vi "ACIR Instrument UI.vi"() -> ()   [LabVIEW 2025, in "ACIR.lvlib" / "ACIR Instrument.lvclass"]
doc: "Copyright 2017 National Instruments Corporation\n\nLicensed under the Apache License, Version 2.0 (the \"License\"); you may not use this file except in compliance with the License. You may obtain a copy of the License at http://www.apache.org/licenses/LICENSE-2.0\nUnless required by applicable law or agreed to in writing, software distributed under the License is distributed on an \"AS IS\" BASIS, WITHOUT WARRANTIES OR CONDITIONS OF ANY KIND, either express or implied. See the License for the specific language governing permissions and limitations under the License."
uses:
  ACIR Instrument.lvclass
  Users/Public/Documents/Sandia National Labs/TSS Plugin/CEF.lvlibp/Node/NodeRef.ctl
  Users/Public/Documents/Sandia National Labs/TSS Plugin/CEF.lvlibp/Node/CEF_Node.lvclass
  Users/Public/Documents/Sandia National Labs/TSS Plugin/CEF.lvlibp/Node/mainQref.ctl
  Users/Public/Documents/Sandia National Labs/TSS Plugin/CEF.lvlibp/Node/UserEventRef.ctl
  Users/Public/Documents/Sandia National Labs/TSS Plugin/Abstract Engine.lvlibp/Instrument configuration/Default Instrument.ctl
  ACIR configuration/ACIR Instrument Setting.ctl
  C:/Users/Public/Documents/Sandia National Labs/TSS Plugin/CEF.lvlibp/Node/CEF_Node.lvclass
  ACIR Instrument.lvclass/ACIR Instrument.ctl
  ACIR configuration/ACIR configuration.lvclass/ACIR configuration.ctl
  ACIR configuration/Read ACIR Setting.vi
  ACIR configuration/Write ACIR Setting.vi
  <vilib>/Utility/error.llb/Trim Whitespace One-Sided.vi
  ACIR configuration/ACIR configuration.lvclass
  C:/Users/Public/Documents/Sandia National Labs/TSS Plugin/Abstract Engine.lvlibp/Instrument configuration/Instrument configuration.lvclass
  Users/Public/Documents/Sandia National Labs/TSS Plugin/Abstract Engine.lvlibp/Instrument configuration/Read Instrument Setting.vi
  Users/Public/Documents/Sandia National Labs/TSS Plugin/Abstract Engine.lvlibp/Instrument configuration/Write Instrument Setting.vi
  Users/Public/Documents/Sandia National Labs/TSS Plugin/Abstract Engine.lvlibp/Instrument configuration/Instrument configuration.lvclass
panel:
  in  "ACIR":cluster{"Default":T1, "Setting":T2}={"Default"={"Type"="NI Digitizer", "Address"="None", "SW Alias"="None", "Description"="* Type = Class\n\n** Concrete = Specific  Device\nConcreate should be same with Type\n ", "Enabled"=TRUE}, "Setting"={"Frequency"=0.0, "Range"="100m Ohm", "Measurements"="Impedence"}} {"Setting"."Frequency" format="%#_6p"}
  in  "user event":T3
  in  "main queue":T4
  in  "node ref":T5
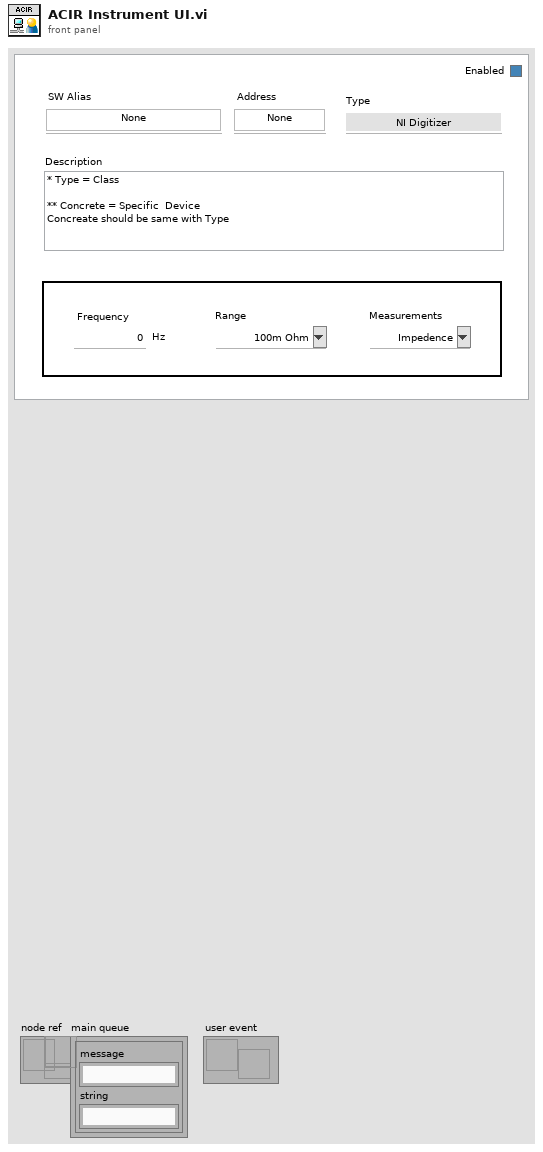
[diagram p1: front panel]
types:
  T1 = typedef "Abstract Engine.lvlibp/Instrument configuration.lvclass/Default Instrument.ctl" = cluster{"Type":string, "Address":string, "SW Alias":string, "Description":string, "Enabled":bool}
  T2 = typedef "ACIR.lvlib/ACIR configuration.lvclass/ACIR Instrument Setting.ctl" = cluster{"Frequency":dbl, "Range":string, "Measurements":string}
  T3 = typedef "CEF.lvlibp/CEF_Node.lvclass/UserEventRef.ctl" = refnum<user-event>
  T4 = typedef "CEF.lvlibp/CEF_Node.lvclass/mainQref.ctl" = refnum<queue>
  T5 = typedef "CEF.lvlibp/CEF_Node.lvclass/NodeRef.ctl" = refnum<data-value>
  T6 = cluster{"Instrument Setting":T1, "ACIR Setting":T2}
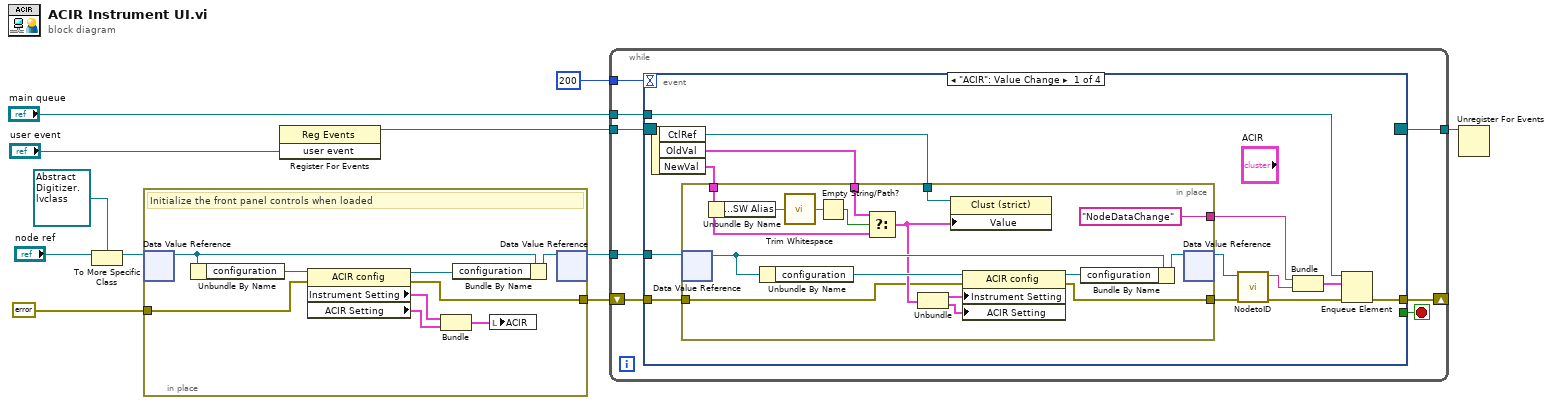
[diagram p0: block diagram]
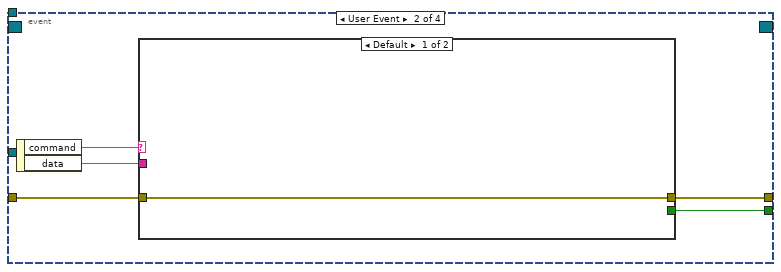
[diagram p2: hidden frame]
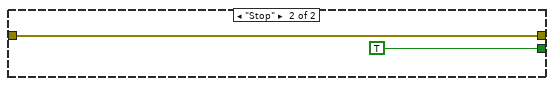
[diagram p3: hidden frame]
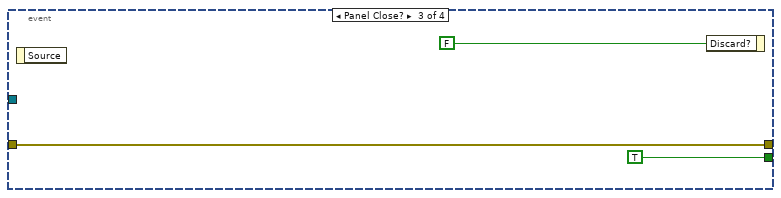
[diagram p4: hidden frame]
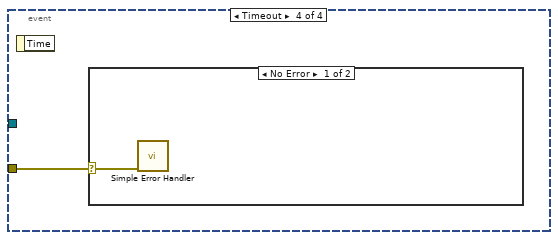
[diagram p5: hidden frame]
diagram:
  n1 = To More Specific Class(target class=refnum<data-value> refnum ("data value reference"), reference="node ref") -> (specific class reference=w4:refnum<data-value>)  [unwired: 1 in, 1 out]
  n2 = in-place {
    in-place-border: errorcluster {"status"=FALSE, "code"=0, "source"=""} ("error out") -> [w17]
    in-place-border: [w16] -> w2
    # "Initialize the front panel controls when loaded"
    n3 = in-place-dvr #1(w4) -> (w18:refnum<class "ACIR Instrument.lvclass">)  [unwired: 1 out]
    n4 = Unbundle By Name(w18) -> ("configuration"=w19:refnum<class "ACIR configuration.lvclass">)
    n5 = property class="ACIR config"(reference=w19, error in=w17) -> (reference out=w15:refnum<class "ACIR configuration.lvclass">, error out=w16:errorcluster, "Instrument Setting"=w14:T1, "ACIR Setting"=w13:T2)
    n6 = Bundle("Instrument Setting"=w14, "ACIR Setting"=w13) -> (w12:T6)  [unwired: 1 in]
    n7 = Bundle By Name(cluster=w18, "configuration"=w15) -> (w20:refnum<class "ACIR Instrument.lvclass">)
    n8 = local write "ACIR"(w12) -> ()
    n9 = in-place-dvr #1(w20) -> (w9:refnum<data-value>)  [unwired: 1 out]
  }
  n10 = register-events("user event") -> (reference out=w6:refnum<event-registration>)  [unwired: 2 in, 1 out]
  n11 = while {
    tunnel: w9 -> [w28]
    tunnel: "main queue" -> [w25]
    tunnel: [w24] -> w7
    tunnel: w6 -> [w23]
    shift-right: [w26] -> _
    shift-left: w2 -> [w22]
    tunnel: 200 -> [w21]
    stop <- w27 stop-if-true
    n12 = event shown="[0] \"ACIR\": Value Change" {
      selector: w23 -> [_ _ _ _]
      dyn-events: [_ _ _ _] -> w24
      timeout: w21 -> [_ _ _ _]
      tunnel: w28 -> [w39 _ _ _]
      tunnel: [_ w60 TRUE _] -> w27
      tunnel: [w41 w58 w66 _] -> w26
      tunnel: w25 -> [w40 _ _ _]
      tunnel: w22 -> [w34 w59 w66 w69]
      event "ACIR": Value Change {
        n13 = event-data() -> ("CtlRef"=w36:refnum<vi>, "OldVal"=w37:cluster{"Default":T1, "Setting":T2}, "NewVal"=w35:cluster{"Default":T1, "Setting":T2})  [unwired: 1 in]
        n14 = in-place {
          in-place-border: [w54] -> w30
          in-place-border: w37 -> [w53]
          in-place-border: w36 -> [w52]
          in-place-border: w35 -> [w49]
          in-place-border: w34 -> [w43]
          in-place-border: ["NodeDataChange" ("Message Name")] -> w33
          n15 = in-place-dvr #2(w39) -> (w57:refnum<class "ACIR Instrument.lvclass">)  [unwired: 1 out]
          n16 = Unbundle By Name(w49) -> ("Default.SW Alias"=w51:string)
          n17 = Unbundle By Name(w57) -> ("configuration"=w47:refnum<class "ACIR configuration.lvclass">)
          n18 = call <vilib>:"Trim Whitespace.vi"("string"=w51) -> ("trimmed string"=w48:string)  [unwired: 1 in]
          n19 = Empty String/Path?(string/path=w48) -> (empty?=w50:bool)
          n20 = Select(t=w53, s=w50, f=w49) -> (s? t:f=w46:cluster{"Default":T1, "Setting":T2})
          n21 = Unbundle(w46) -> ("Default"=w45:T1, "Setting"=w44:T2)
          n22 = property class="Clust (strict)"(reference=w52, "Value"=w46) -> ()  [unwired: 1 in, 2 out]
          n23 = property class="ACIR config"(reference=w47, error in=w43, "Instrument Setting"=w45, "ACIR Setting"=w44) -> (reference out=w55:refnum<class "ACIR configuration.lvclass">, error out=w54:errorcluster)
          n24 = Bundle By Name(cluster=w57, "configuration"=w55) -> (w56:refnum<class "ACIR Instrument.lvclass">)
          n25 = in-place-dvr #2(w56) -> (w38:refnum<data-value>)  [unwired: 1 out]
        }
        n26 = call "NodetoID.vi"("error in"=w30, "node ref"=w38) -> ("error out"=w29:errorcluster, "ID"=w31:string)  [unwired: 8 in]
        n27 = Bundle("Message Name"=w33, "ID"=w31) -> (w32:cluster{"Message Name":string, "ID":string})  [unwired: 1 in]
        n28 = Enqueue Element(queue=w40, element=w32, error in (no error)=w29) -> (error out=w41:errorcluster)  [unwired: 1 in, 2 out]
      }
      event User Event {
        n29 = event-data() -> ("command"=w62:string, "data"=w61:string)  [unwired: 1 in]
        n30 = case shown="Default" w62 {
          tunnel: w61 -> [_ _]
          tunnel: [_ TRUE] -> w60
          tunnel: w59 -> [w63 w64]
          tunnel: [w63 w64] -> w58
          frame Default {
          }
          frame "Stop" {
          }
        }
      }
      event Panel Close? {
        n31 = event-data() -> ()  [unwired: 1 in, 1 out]
        n32 = event-data("Discard?"=FALSE) -> ()  [unwired: 1 in, 1 out]
      }
      event Timeout {
        n33 = event-data() -> ()  [unwired: 1 in, 1 out]
        n34 = case shown="No Error" w69 {
          selector: w69 -> [w70 _]
          frame No Error {
            n35 = call <vilib>:"Simple Error Handler.vi"("error in (no error)"=w70) -> ()  [unwired: 4 in, 5 out]
          }
          frame Error {
          }
        }
      }
    }
  }
  n36 = Unregister For Events(event registration refnum=w7) -> ()  [unwired: 1 in, 1 out]
